vi "Create RSASignaturePadding.vi"(8 "error in (no error)":errorcluster, 11 "RSASignaturePadding":T1) -> (0 "error out":errorcluster, 3 "RSASignaturePadding out":refnum<k24>)   [LabVIEW 2021, in "dotNET Crypto Asymmetric Encryption.lvlib"]
doc: "Creates an RSASignaturePadding object - ensure that the object is closed to avoid a reference leak."
uses:
  dotNET Crypto Asymmetric Encryption.lvlib
  RSASignaturePadding.ctl
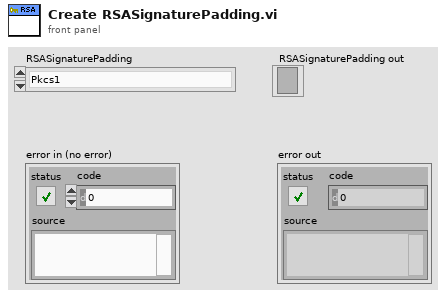
[diagram p1: front panel]
types:
  T1 = typedef "dotNET Crypto Asymmetric Encryption.lvlib/RSASignaturePadding.ctl" = enum16{"Pkcs1", "Pss"}
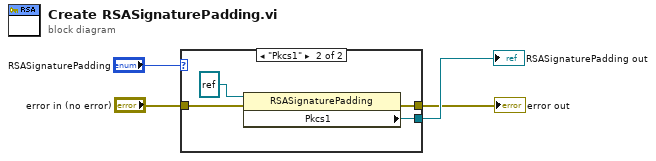
[diagram p0: block diagram]
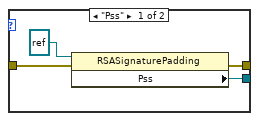
[diagram p2: hidden frame]
diagram:
  n1 = case shown="\"Pkcs1\"" "RSASignaturePadding" {
    tunnel: [w8 w12] -> w3
    tunnel: "error in (no error)" -> [w7 w11]
    tunnel: [w6 w10] -> w1
    frame "Pss" {
      n2 = property class="RSASignaturePadding"(reference=refnum<k24> refnum ("padding"), error in=w7) -> (error out=w6:errorcluster, "Pss"=w8:refnum<k24>)  [unwired: 1 out]
    }
    frame "Pkcs1" {
      n3 = property class="RSASignaturePadding"(reference=refnum<k24> refnum ("padding"), error in=w11) -> (error out=w10:errorcluster, "Pkcs1"=w12:refnum<k24>)  [unwired: 1 out]
    }
  }
  "RSASignaturePadding out" <- w3
  "error out" <- w1
